vi "Keys.vi"(8 "error in (no error)":errorcluster, 11 "Ini Path in":path) -> (0 "error out":errorcluster, 2 "Sections":T1(array[cluster]), 3 "Ini Path out":path)   [LabVIEW 2021, in "Config.lvlib"]
uses:
  Config.lvlib
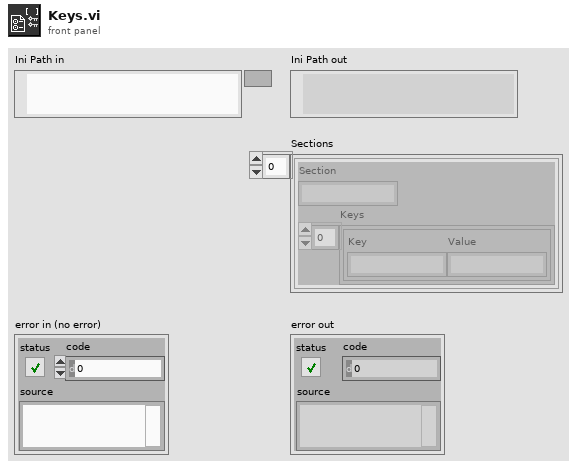
[diagram p1: front panel]
types:
  T1 = cluster{"Section":string, "Keys":cluster{"Key":string, "Value":string}[]}[]
  T2 = cluster{"Section":string, "Keys":cluster{"Key":string, "Value":string}[]}
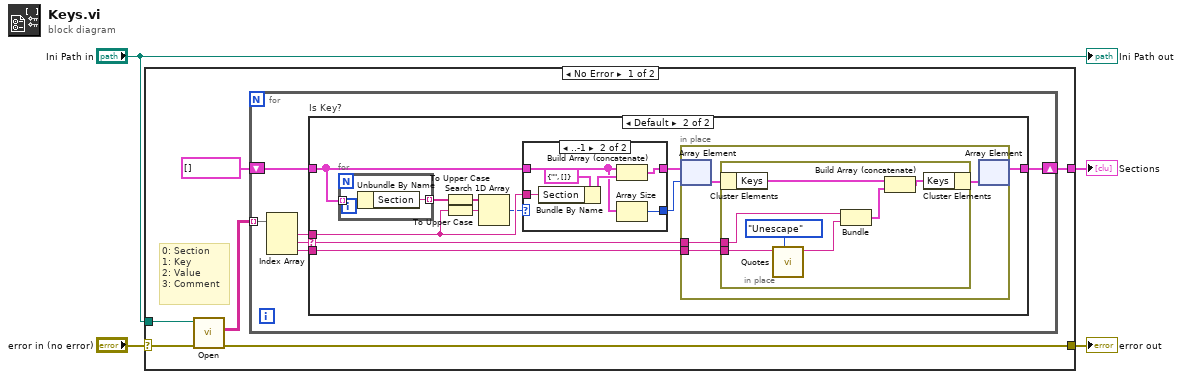
[diagram p0: block diagram]
diagram:
  n1 = case shown="No Error" "error in (no error)" {
    selector: "error in (no error)" -> [w10 w50]
    tunnel: [w9 w50] -> w2
    tunnel: "Ini Path in" -> [w8 _]
    tunnel: [w5 _] -> w1
    frame No Error {
      # "0: Section\n1: Key\n2: Value\n3: Comment"
      n2 = call "Open.vi"("error in (no error)"=w10, "Ini Path in"=w8) -> ("error out"=w9:errorcluster, "skvc out"=w6:string[][])  [unwired: 6 in, 2 out]
      n3 = for {
        tunnel: w6 -> [w14] mode=indexing
        shift-right: [w15] -> w5
        shift-left: T1 [] ("Sections") -> [w16]
        n4 = Index Array(array=w14) -> (element #1=w13:string, element #2=w12:string, element #3=w11:string)  [unwired: 3 in]
        n5 = case "Is Key?" shown="Default" w12 {
          selector: w12 -> [_ w23]
          tunnel: w16 -> [w17 w25]
          tunnel: [w17 w24] -> w15
          tunnel: w13 -> [_ w20]
          tunnel: w11 -> [_ w22]
          frame "" {
          }
          frame Default {
            n6 = for {
              tunnel: w25 -> [w38] mode=indexing
              tunnel: [w37] -> w28 mode=indexing
              n7 = Unbundle By Name(w38) -> ("Section"=w37:string)
            }
            n8 = To Upper Case(1:w28) -> (0:w26:string[])
            n9 = To Upper Case(1:w20) -> (0:w27:string)
            n10 = Search 1D Array(1D array=w26, element=w27) -> (index of element=w19:i32)  [unwired: 1 in]
            n11 = case shown="..-1" w19 {
              selector: w19 -> [w30 _]
              tunnel: w25 -> [w29 w32]
              tunnel: [w29 w36] -> w21
              tunnel: w20 -> [_ w33]
              tunnel: [w30 w31] -> w18
              frame 0.. {
              }
              frame ..-1 {
                n12 = Bundle By Name(cluster=T2 {"Section"="", "Keys"=[]}, "Section"=w33) -> (w34:T2)
                n13 = Build Array (concatenate)(w32, w34) -> (w36:T1)
                n14 = Array Size(array=w32) -> (size(s)=w31:i32)
              }
            }
            n15 = in-place {
              in-place-border: w23 -> [w41]
              in-place-border: w22 -> [w39]
              n16 = in-place-array #1(w21, w18) -> (w42:T2)
              n17 = in-place {
                in-place-border: w41 -> [w47]
                in-place-border: w39 -> [w46]
                n18 = in-place-cluster #2(w42) -> ("Keys"=w49:cluster{"Key":string, "Value":string}[])
                n19 = call "Quotes.vi"("Action"=enum8{"Escape", "Unescape"}."Unescape", "String in"=w46) -> ("String out"=w44:string)  [unwired: 9 in]
                n20 = Bundle(w47, "String out"=w44) -> (w45:cluster{string, "String out":string})  [unwired: 1 in]
                n21 = Build Array (concatenate)(w49, w45) -> (w48:cluster{"Key":string, "String out":string}[])
                n22 = in-place-cluster #2("Keys"=w48) -> (w40:T2)
              }
              n23 = in-place-array #1(w40) -> (w24:T1)  [unwired: 1 out]
            }
          }
        }
      }
    }
    frame Error {
    }
  }
  "error out" <- w2
  "Sections" <- w1
  "Ini Path out" <- "Ini Path in"
